vi "Exp Random.vi"(6 "seed":i32=-1, 7 "reset":bool, 9 "b":dbl=2.0, 10 "a":dbl=1.0, 11 "samples":i32=128) -> (0 "error":i32, 3 "exp random data":dbl[](array[numeric]))   [LabVIEW 2017, in "NI_Gmath.lvlib"]
doc: "Generates random values from a variate X, where X describes the selected distribution type. You must manually select the polymorphic instance to use."
uses:
  <vilib>/gmath/NI_Gmath.lvlib
  <vilib>/gmath/statdist.llb/st_error_code.ctl
panel:
  # "Exp Random"
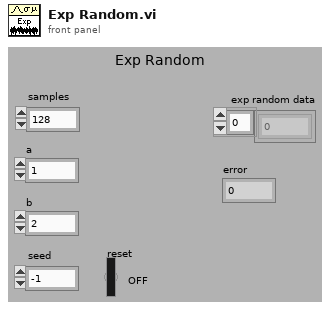
[diagram p1: front panel]
types:
  T1 = typedef "NI_Gmath.lvlib/st_error_code.ctl" = i32
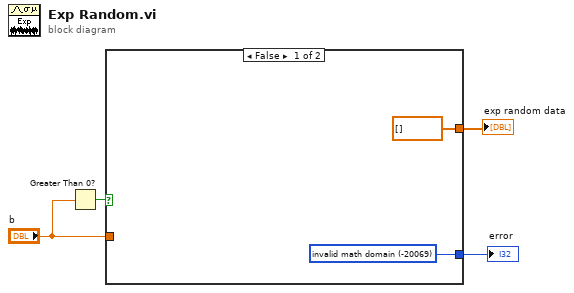
[diagram p0: block diagram]
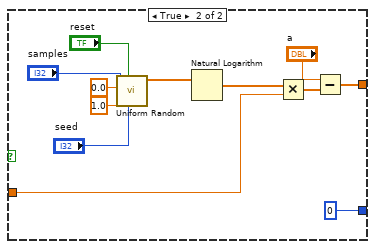
[diagram p2: hidden frame]
diagram:
  n1 = Greater Than 0?(x="b") -> (x > 0?=w4:bool)
  n2 = case shown="False" w4 {
    tunnel: [dbl[] [] w8] -> w2
    tunnel: "b" -> [_ w7]
    tunnel: [w5 0] -> w1
    frame False {
      w5 = T1 -20069 items=["invalid math domain"=-20069, "Fourier interpolation size m >= n"=-20070, "empty array"=-20003] ("stat interp error code")
    }
    frame True {
      n3 = call <vilib>:"Uniform Random.vi"("seed"="seed", "reset"="reset", "xmax"=1.0, "xmin"=0.0, "samples"="samples") -> ("uniform random data"=w10:dbl[])  [unwired: 5 in, 1 out]
      n4 = Natural Logarithm(1:w10) -> (0:w9:dbl[])
      n5 = Multiply(x=w9, y=w7) -> (x*y=w16:dbl[])
      n6 = Subtract(x="a", y=w16) -> (x-y=w8:dbl[])
    }
  }
  "error" <- w1
  "exp random data" <- w2
